vi "Find Fiducial.vi"(4 "Field of View":cluster{"fieldOfViewX":sgl, "fieldOfViewY":sgl}, 5 "Shrink Factor":i32=1, 6 "debug":bool, 7 "Log File Directory":string, 8 "error in":errorcluster, 9 "Method Parameters":variant, 10 "Method Name":string, 11 "Image":T2) -> (0 "error out":errorcluster, 2 "Fiducials":T1(array[cluster]))   [LabVIEW 2017, in "Vision.lvlib"]
uses:
  Vision.lvlib
  <vilib>/vision/Image Controls.llb/IMAQ Image.ctl
  find_circles parameters.ctl
  find_patches parameters.ctl
  find_rects_parameters.ctl
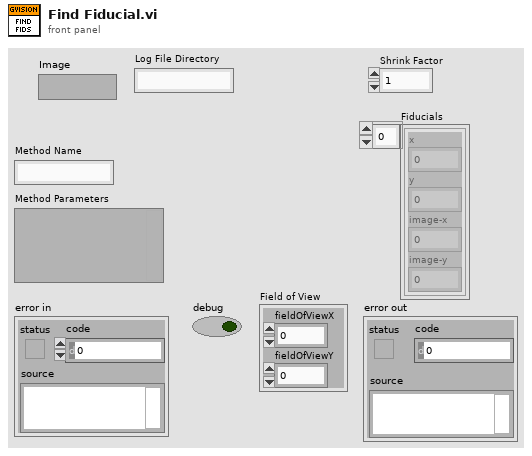
[diagram p1: front panel]
types:
  T1 = cluster{"x":dbl, "y":dbl, "image-x":dbl, "image-y":dbl}[]
  T2 = typedef "IMAQ Image.ctl" = refnum<image>
  T3 = typedef "Vision.lvlib/find_circles parameters.ctl" = cluster{"minRadius":sgl, "maxRadius":sgl, "houghGradientParam1":i32, "houghGradientParam2":i32}
  T4 = cluster{"x":dbl, "y":dbl, "image-x":dbl, "image-y":dbl}
  T5 = typedef "Vision.lvlib/find_patches parameters.ctl" = cluster{"dilateSize":i32, "sizeMin":sgl, "sizeMax":sgl, "aspectRatioMin":sgl, "aspectRatioMax":sgl, "colorGroups":i32}
  T6 = typedef "Vision.lvlib/find_rects_parameters.ctl" = cluster{"nominalWidth":sgl, "nominalHeight":sgl, "tolerance":sgl, "pointSelect":sgl}
  T7 = cluster{"x":dbl, "y":dbl, "radius":dbl, "image-x":dbl, "image-y":dbl}[]
  T8 = cluster{"x":dbl, "y":dbl, "aspect ratio":dbl, "size":dbl, "image-x":dbl, "image-y":dbl}[]
  T9 = cluster{"x":dbl, "y":dbl, "width":dbl, "height":dbl, "angle":dbl, "image-x":dbl, "image-y":dbl}[]
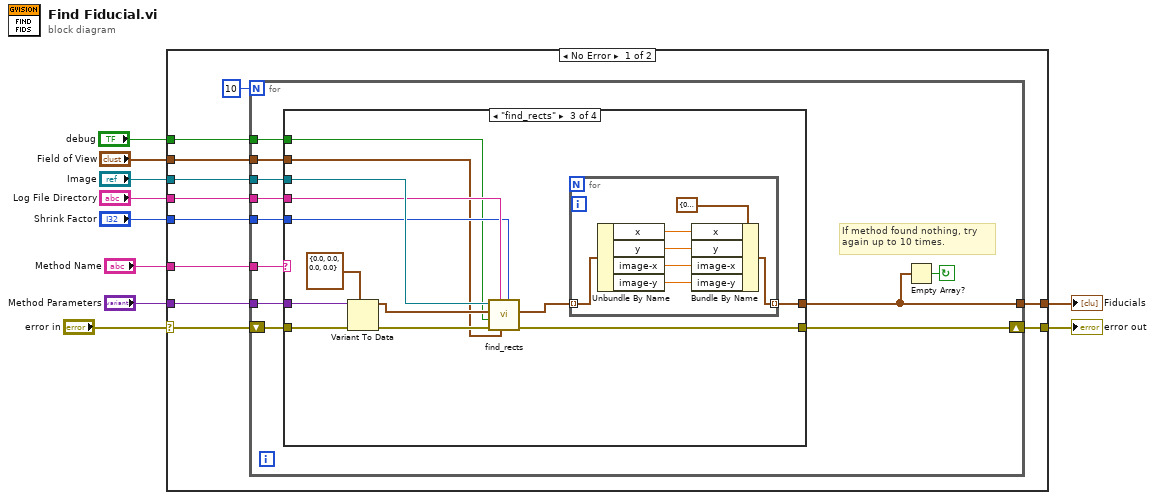
[diagram p0: block diagram]
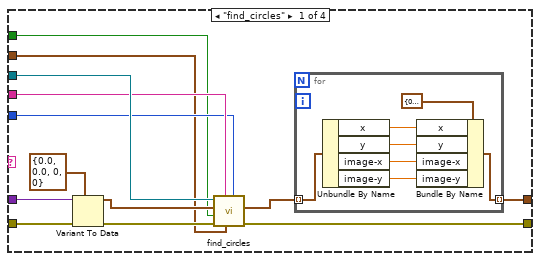
[diagram p2: hidden frame]
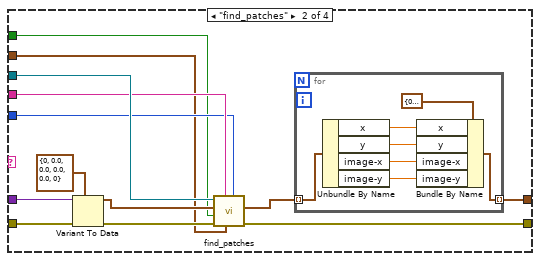
[diagram p3: hidden frame]
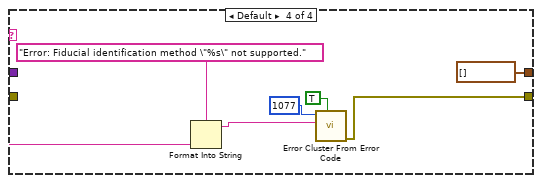
[diagram p4: hidden frame]
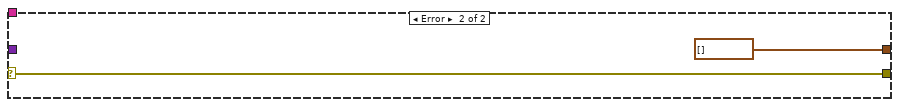
[diagram p5: hidden frame]
diagram:
  n1 = case shown="No Error" "error in" {
    selector: "error in" -> [w19 w101]
    tunnel: [w12 w101] -> w9
    tunnel: "Method Name" -> [w21 _]
    tunnel: "Method Parameters" -> [w20 _]
    tunnel: "Image" -> [w18 _]
    tunnel: "Log File Directory" -> [w17 _]
    tunnel: "Shrink Factor" -> [w16 _]
    tunnel: "Field of View" -> [w15 _]
    tunnel: "debug" -> [w14 _]
    tunnel: [w13 T1 []] -> w1
    frame No Error {
      n2 = for {
        N: 10 -> [_]
        tunnel: w21 -> [w32]
        tunnel: w20 -> [w31]
        tunnel: w18 -> [w29]
        tunnel: w17 -> [w28]
        tunnel: w16 -> [w27]
        tunnel: w15 -> [w26]
        tunnel: w14 -> [w25]
        tunnel: [w23] -> w13
        shift-right: [w24] -> w12
        shift-left: w19 -> [w30]
        stop <- w22 continue-if-true
        # "If method found nothing, try\nagain up to 10 times."
        n3 = case shown="\"find_rects\"" w32 {
          selector: w32 -> [_ _ _ w97]
          tunnel: w31 -> [w45 w65 w85 _]
          tunnel: w30 -> [w42 w63 w83 _]
          tunnel: w29 -> [w40 w61 w81 _]
          tunnel: w28 -> [w39 w60 w80 _]
          tunnel: w27 -> [w38 w59 w79 _]
          tunnel: w26 -> [w36 w57 w77 _]
          tunnel: w25 -> [w37 w58 w78 _]
          tunnel: [w34 w55 w75 T1 []] -> w23
          tunnel: [w33 w53 w74 w93] -> w24
          frame "find_circles" {
            n4 = Variant To Data(error in=w42, type=T3 {"minRadius"=0.0, "maxRadius"=0.0, "houghGradientParam1"=0, "houghGradientParam2"=0} ("find_circles parameters"), Variant=w45) -> (data=w43:T3, error out=w41:errorcluster)
            n5 = call "find_circles.vi"("shrinkFactor"=w38, "Field of View"=w36, "logFileDir"=w39, "error in"=w41, "debug"=w37, "find_circles parameters"=w43, "Image"=w40) -> ("error out"=w33:errorcluster, "Circles"=w35:T7)  [unwired: 3 in]
            n6 = for {
              tunnel: w35 -> [w52] mode=indexing
              tunnel: [w46] -> w34 mode=indexing
              n7 = Unbundle By Name(w52) -> ("x"=w50:dbl, "y"=w49:dbl, "image-x"=w48:dbl, "image-y"=w47:dbl)
              n8 = Bundle By Name(cluster=T4 {"x"=0.0, "y"=0.0, "image-x"=0.0, "image-y"=0.0}, "x"=w50, "y"=w49, "image-x"=w48, "image-y"=w47) -> (w46:T4)
            }
          }
          frame "find_patches" {
            n9 = Variant To Data(error in=w63, type=T5 {"dilateSize"=0, "sizeMin"=0.0, "sizeMax"=0.0, "aspectRatioMin"=0.0, "aspectRatioMax"=0.0, "colorGroups"=0} ("find_patches parameters"), Variant=w65) -> (data=w64:T5, error out=w62:errorcluster)
            n10 = call "find_patches.vi"("Shrink Factor"=w59, "Field of View"=w57, "Log File Directory"=w60, "error in"=w62, "debug"=w58, "find_patches parameters"=w64, "Image"=w61) -> ("error out"=w53:errorcluster, "Patches"=w56:T8)  [unwired: 3 in]
            n11 = for {
              tunnel: w56 -> [w72] mode=indexing
              tunnel: [w66] -> w55 mode=indexing
              n12 = Unbundle By Name(w72) -> ("x"=w70:dbl, "y"=w69:dbl, "image-x"=w68:dbl, "image-y"=w67:dbl)
              n13 = Bundle By Name(cluster=T4 {"x"=0.0, "y"=0.0, "image-x"=0.0, "image-y"=0.0}, "x"=w70, "y"=w69, "image-x"=w68, "image-y"=w67) -> (w66:T4)
            }
          }
          frame "find_rects" {
            n14 = Variant To Data(error in=w83, type=T6 {"nominalWidth"=0.0, "nominalHeight"=0.0, "tolerance"=0.0, "pointSelect"=0.0} ("find_patches parameters"), Variant=w85) -> (data=w84:T6, error out=w82:errorcluster)
            n15 = call "find_rects.vi"("shrinkFactor"=w79, "Field of View"=w77, "logFileDir"=w80, "error in"=w82, "debug"=w78, "find_patches parameters"=w84, "Image"=w81) -> ("error out"=w74:errorcluster, "rects"=w76:T9)  [unwired: 3 in]
            n16 = for {
              tunnel: w76 -> [w92] mode=indexing
              tunnel: [w86] -> w75 mode=indexing
              n17 = Unbundle By Name(w92) -> ("x"=w90:dbl, "y"=w89:dbl, "image-x"=w88:dbl, "image-y"=w87:dbl)
              n18 = Bundle By Name(cluster=T4 {"x"=0.0, "y"=0.0, "image-x"=0.0, "image-y"=0.0}, "x"=w90, "y"=w89, "image-x"=w88, "image-y"=w87) -> (w86:T4)
            }
          }
          frame Default {
            n19 = Format Into String(format string="Error: Fiducial identification method \"%s\" not supported.", w97) -> (resulting string=w96:string)  [unwired: 2 in, 1 out]
            n20 = call <vilib>:"Error Cluster From Error Code.vi"("show call chain? (False)"=TRUE, "error message (\"\")"=w96, "error code (0)"=1077) -> ("error out"=w93:errorcluster)  [unwired: 6 in]
          }
        }
        n21 = Empty Array?(array=w23) -> (empty?=w22:bool)
      }
    }
    frame Error {
    }
  }
  "error out" <- w9
  "Fiducials" <- w1
